vi "MovePosition.vi"(8 "error in (no error)":errorcluster, 10 "Position Delta":cluster{"X":sgl, "Y":sgl, "Z":sgl}, 11 "3D Scene in":refnum<class "3D Scene.lvclass">) -> (0 "error out":errorcluster, 3 "3D Scene out":refnum<class "3D Scene.lvclass">)   [LabVIEW 2015, in "3D Scene.lvclass"]
uses:
  3D Scene.lvclass
  3D Scene.lvclass/3D Scene.ctl
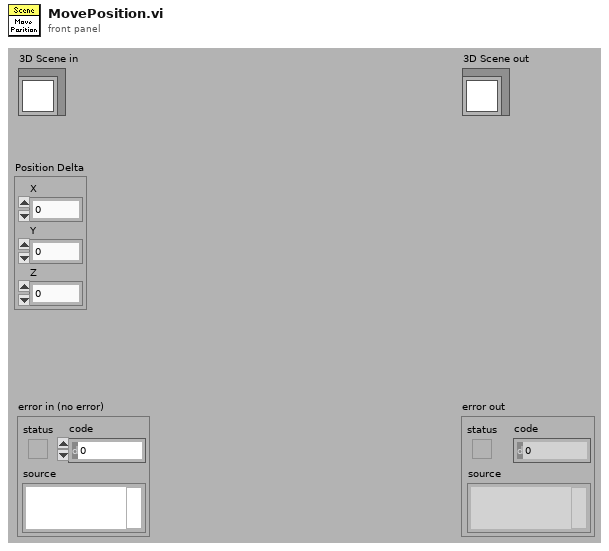
[diagram p1: front panel]
types:
  T1 = typedef "3D Point.ctl" = cluster{"X":sgl, "Y":sgl, "Z":sgl}
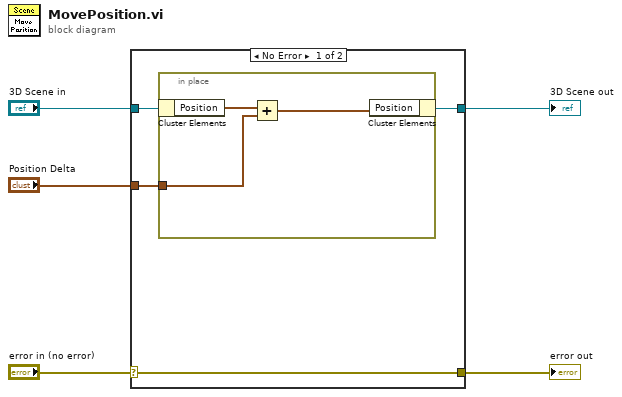
[diagram p0: block diagram]
diagram:
  n1 = case shown="No Error" "error in (no error)" {
    selector: "error in (no error)" -> [w9 w14]
    tunnel: [w9 w14] -> w4
    tunnel: [w7 w13] -> w2
    tunnel: "3D Scene in" -> [w8 w13]
    tunnel: "Position Delta" -> [w6 _]
    frame No Error {
      n2 = in-place {
        in-place-border: w6 -> [w11]
        n3 = in-place-cluster #1(w8) -> ("Position"=w12:T1)
        n4 = Add(x=w12, y=w11) -> (x+y=w10:T1)
        n5 = in-place-cluster #1("Position"=w10) -> (w7:refnum<class "3D Scene.lvclass">)
      }
    }
    frame Error {
    }
  }
  "error out" <- w4
  "3D Scene out" <- w2
